vi "reset_test.vi"() -> ()   [LabVIEW 2017]
panel:
  out "Numeric":i32
  out "error out 2":errorcluster
  in  "SoftTriggerEnable":bool=TRUE
  in  "address":string="192.168.10.20"
  out "error out":errorcluster
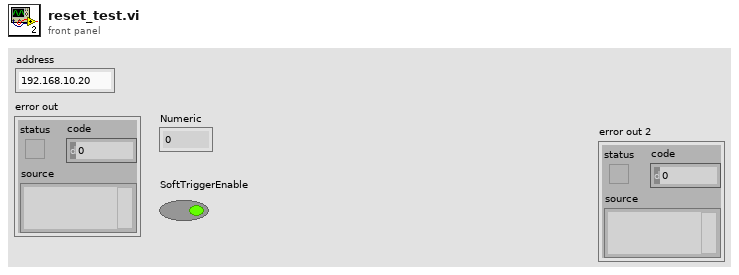
[diagram p1: front panel]
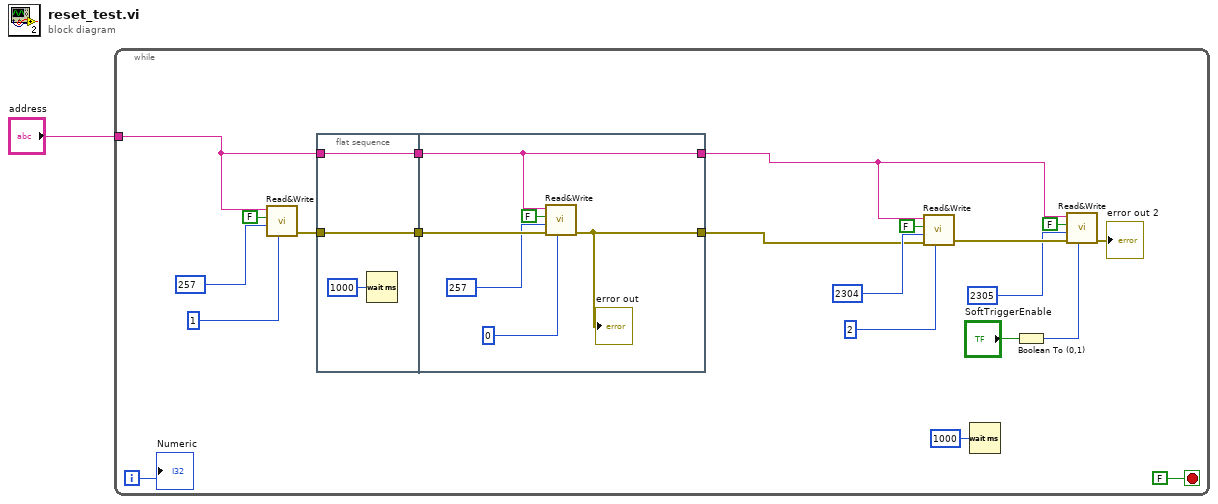
[diagram p0: block diagram]
diagram:
  n1 = while {
    tunnel: "address" -> [w20]
    i -> [w2]
    stop <- FALSE stop-if-true
    n2 = call "Read&Write.vi"("In"=u8 1, "Address"=u32 257, "Read (TRUE)"=FALSE, "address"=w20) -> ("error out"=w19:errorcluster)  [unwired: 6 in, 1 out]
    n3 = flat-sequence {
      tunnel: w19 -> [w24]
      tunnel: w20 -> [w25]
      tunnel: [w25] -> w22
      tunnel: [w24] -> w21
      tunnel: w22 -> [w27]
      tunnel: w21 -> [w31]
      tunnel: [w27] -> w6
      tunnel: [w26] -> w5
      frame #0 {
        n4 = Wait (ms)(milliseconds to wait=u32 1000) -> ()  [unwired: 1 out]
      }
      frame #1 {
        n5 = call "Read&Write.vi"("In"=u8 0, "error in (no error)"=w31, "Address"=u32 257, "Read (TRUE)"=FALSE, "address"=w27) -> ("error out"=w26:errorcluster)  [unwired: 5 in, 1 out]
        "error out" <- w26
      }
    }
    n6 = call "Read&Write.vi"("In"=u8 2, "error in (no error)"=w5, "Address"=u32 2304, "Read (TRUE)"=FALSE, "address"=w6) -> ("error out"=w15:errorcluster)  [unwired: 5 in, 1 out]
    n7 = Wait (ms)(milliseconds to wait=u32 1000) -> ()  [unwired: 1 out]
    n8 = Boolean To (0,1)(Boolean="SoftTriggerEnable") -> (0, 1=w8:i16)
    n9 = call "Read&Write.vi"("In"=w8, "error in (no error)"=w15, "Address"=u32 2305, "Read (TRUE)"=FALSE, "address"=w6) -> ("error out"=→"error out 2":errorcluster)  [unwired: 5 in, 1 out]
    "Numeric" <- w2
  }
